vi "Camera and voice coil synchronization.vi"() -> ()   [LabVIEW 2020]
uses:
  <vilib>/DAQmx/write.llb/DAQmx Write (Analog Wfm 1Chan NSamp).vi
  <vilib>/DAQmx/read.llb/DAQmx Read (Analog Wfm 1Chan NSamp).vi
  <vilib>/DAQmx/create/channels.llb/DAQmx Create Channel (AO-Voltage-Basic).vi
  <vilib>/DAQmx/configure/timing.llb/DAQmx Timing (Sample Clock).vi
  <vilib>/DAQmx/configure/trigger.llb/DAQmx Start Trigger (Digital Edge).vi
  <vilib>/DAQmx/create/channels.llb/DAQmx Create Channel (AI-Voltage-Basic).vi
  <vilib>/DAQmx/miscellaneous.llb/DAQmx Fill In Error Info.vi
  <vilib>/measure/NI_MABase.lvlib
  <resource>/objmgr/daqmx.rc
panel:
  out "number of samples written per channel":u32
  out "Waveform Graph 2":waveform(dbl)(graph)
  out "Waveform Graph":waveform(dbl)(graph)
  in  "stop":bool
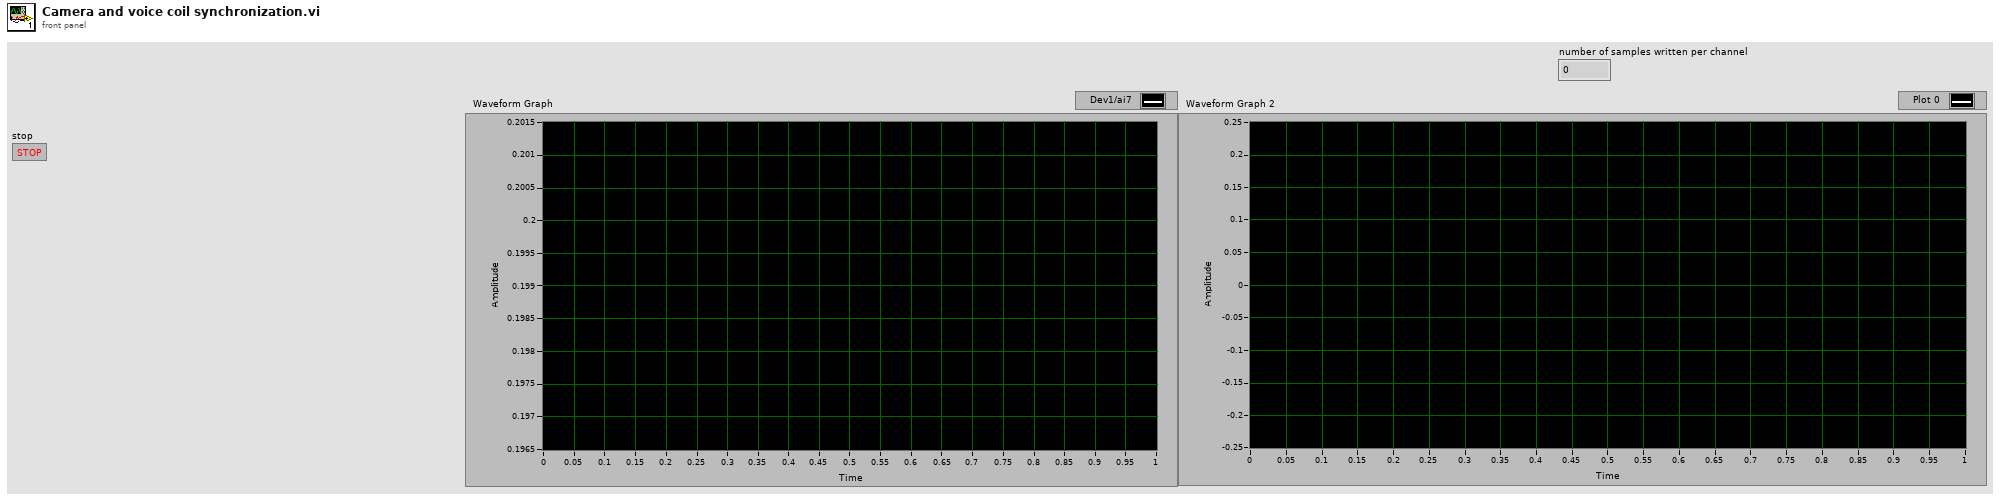
[diagram p1: front panel]
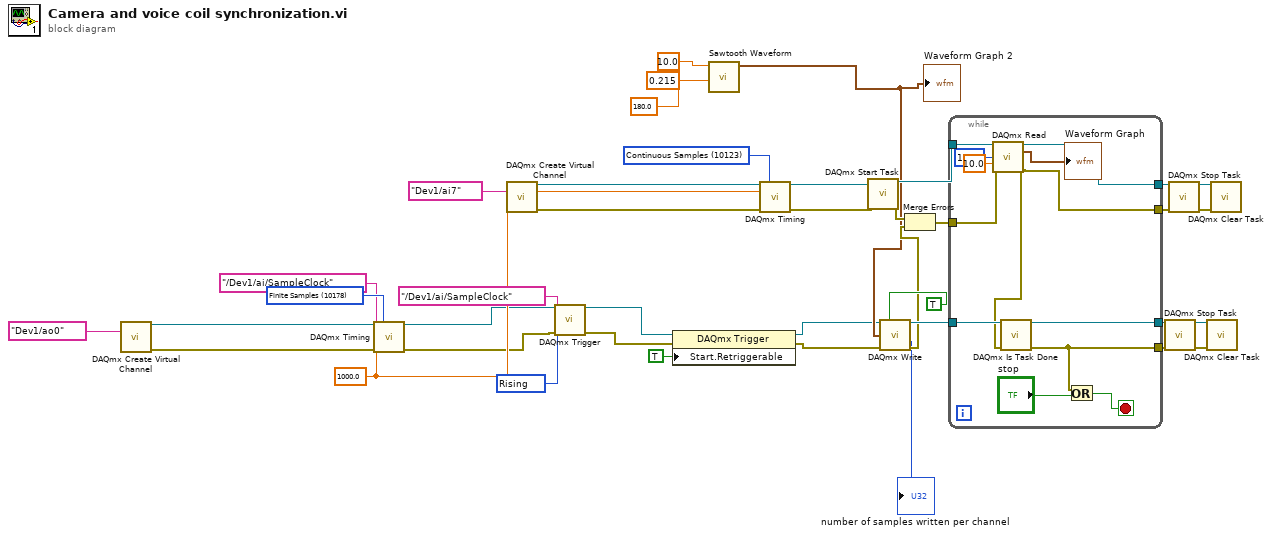
[diagram p0: block diagram]
diagram:
  w8 = 10280 items=["Rising"=10280, "Falling"=10171] ("edge")
  w11 = 1000.0 ("rate")
  w28 = 10178 items=["Finite Samples"=10178, "Continuous Samples"=10123, "Hardware Timed Single Point"=12522] ("sample mode")
  w29 = 10123 items=["Finite Samples"=10178, "Continuous Samples"=10123, "Hardware Timed Single Point"=12522] ("sample mode")
  n1 = call-poly <vilib>:"DAQmx Create Virtual Channel.vi"("physical channels"=tag "Dev1/ao0") -> ("task out"=w37:refnum<k21>, "error out"=w36:errorcluster)  [unwired: 13 in]
  n2 = call-poly <vilib>:"DAQmx Timing.vi"("task/channels in"=w37, "sample mode"=w28, "rate"=w11, "source"=tag "/Dev1/ai/SampleClock", "error in"=w36) -> ("task out"=w10:refnum<k21>, "error out"=w9:errorcluster)  [unwired: 9 in]
  n3 = call-poly <vilib>:"DAQmx Create Virtual Channel.vi"("physical channels"=tag "Dev1/ai7") -> ("task out"=w31:refnum<k21>, "error out"=w30:errorcluster)  [unwired: 13 in]
  n4 = call-poly <vilib>:"DAQmx Trigger.vi"("task/channels in"=w10, "source"=tag "/Dev1/ai/SampleClock", "edge"=w8, "error in"=w9) -> ("task out"=w5:refnum<k21>, "error out"=w3:errorcluster)  [unwired: 10 in]
  n5 = property class="DAQmx Trigger"(reference=w5, error in=w3, "Start.Retriggerable"=TRUE) -> (reference out=w4:refnum<k21>, error out=w2:errorcluster)
  n6 = call <vilib>:"Sawtooth Waveform.vi"("phase"=180.0, "amplitude"=0.215, "frequency"=10.0) -> ("signal out"=w13:waveform(dbl))  [unwired: 7 in, 1 out]
  "Waveform Graph 2" <- w13
  n7 = call-poly <vilib>:"DAQmx Timing.vi"("task/channels in"=w31, "sample mode"=w29, "rate"=w11, "error in"=w30) -> ("task out"=w26:refnum<k21>, "error out"=w25:errorcluster)  [unwired: 10 in]
  n8 = call <vilib>:"DAQmx Start Task.vi"("task/channels in"=w26, "error in"=w25) -> ("task out"=w24:refnum<k21>, "error out"=w23:errorcluster)  [unwired: 12 in]
  n9 = call-poly <vilib>:"DAQmx Write.vi"("task/channels in"=w4, "auto start"=TRUE, "data"=w13, "error in"=w2) -> ("task out"=w35:refnum<k21>, "number of samples written per channel"=→"number of samples written per channel":u32, "error out"=w22:errorcluster)  [unwired: 9 in]
  n10 = Merge Errors(w23, w22) -> (w21:errorcluster)
  n11 = while {
    tunnel: w24 -> [w50]
    tunnel: w21 -> [w49]
    tunnel: [w46] -> w20
    tunnel: w35 -> [w52]
    tunnel: [w51] -> w34
    tunnel: [w48] -> w19
    tunnel: [w47] -> w18
    stop <- w44 stop-if-true
    n12 = call-poly <vilib>:"DAQmx Read.vi"("task/channels in"=w50, "number of samples per channel"=1000, "timeout"=10.0, "error in"=w49) -> ("task out"=w48:refnum<k21>, "data"=→"Waveform Graph":waveform(dbl), "error out"=w47:errorcluster)  [unwired: 9 in]
    n13 = call <vilib>:"DAQmx Is Task Done.vi"("task/channels in"=w52, "error in"=w47) -> ("task out"=w51:refnum<k21>, "error out"=w46:errorcluster)  [unwired: 11 in, 1 out]
    n14 = Or(x=w46, y="stop") -> (x .or. y?=w44:bool)
  }
  n15 = call <vilib>:"DAQmx Stop Task.vi"("task/channels in"=w34, "error in"=w20) -> ("task out"=w38:refnum<k21>, "error out"=w39:errorcluster)  [unwired: 12 in]
  n16 = call <vilib>:"DAQmx Stop Task.vi"("task/channels in"=w19, "error in"=w18) -> ("task out"=w32:refnum<k21>, "error out"=w33:errorcluster)  [unwired: 12 in]
  n17 = call <vilib>:"DAQmx Clear Task.vi"("task in"=w38, "error in"=w39) -> ()  [unwired: 13 in, 1 out]
  n18 = call <vilib>:"DAQmx Clear Task.vi"("task in"=w32, "error in"=w33) -> ()  [unwired: 13 in, 1 out]
